vi "LoadConfig.vi"(8 "error in (no error)":errorcluster, 11 "EpiWrapper in":refnum<class "EpiWrapper.lvclass">) -> (0 "error out":errorcluster, 3 "EpiWrapper out":refnum<class "EpiWrapper.lvclass">)   [LabVIEW 2012, in "EpiWrapper.lvclass"]
uses:
  EpiWrapper.lvclass
  <vilib>/xml/Load XML File.vi
  <vilib>/xml/Close Reference(Node).vi
  <vilib>/xml/Close Reference(NdList).vi
  <resource>/objmgr/DOMUserDefRef.rc
  <vilib>/xml/NI_XML.lvlib
panel:
  out "Array":cluster{"IntTime":string, "Samples":string}[](array[cluster])
  out "Parse Errors":string
  out "XML File Path":path
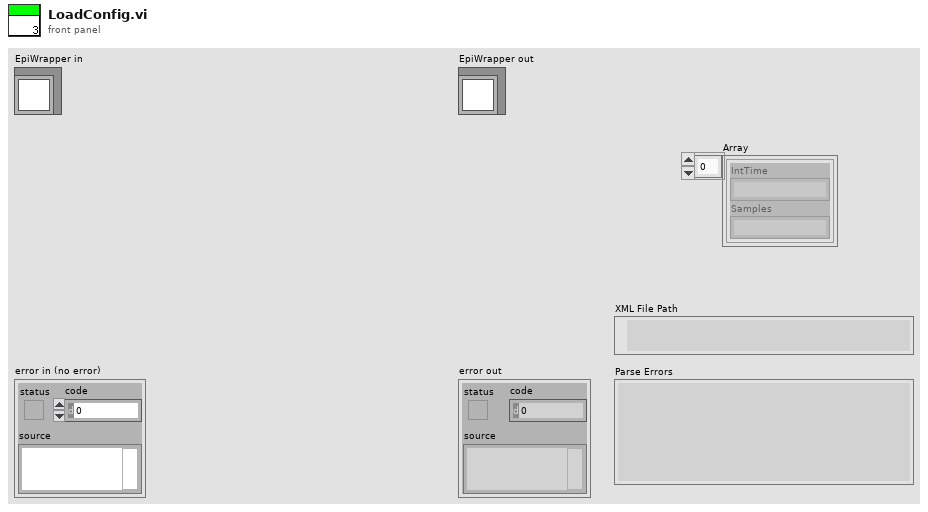
[diagram p1: front panel]
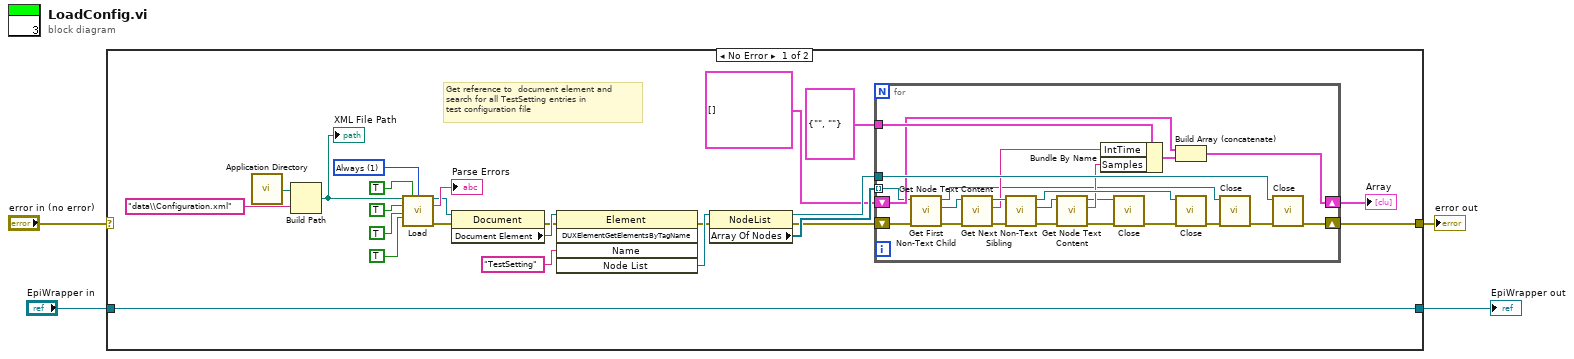
[diagram p0: block diagram]
diagram:
  n1 = case shown="No Error" "error in (no error)" {
    selector: "error in (no error)" -> [_ w53]
    tunnel: "EpiWrapper in" -> [w5 w52]
    tunnel: [w7 w53] -> w2
    tunnel: [w5 w52] -> w1
    frame No Error {
      w25 = 1 items=["Never", "Always", "Auto"] ("Validate On Load")
      # "Get reference to  document element and\nsearch for all TestSetting entries in \ntest configuration file"
      n2 = call <vilib>:"Application Directory.vi"() -> ("Application Directory"=w6:path)
      n3 = Build Path(base path=w6, name or relative path="data\\Configuration.xml") -> (appended path=w15:path)
      "XML File Path" <- w15
      n4 = call-poly <vilib>:"Load.vi"("path to XML document"=w15, "preserve whitespace (True)"=TRUE ("Preserve Whitespace"), "validate on load (Auto)"=w25, "process namespaces (False)"=TRUE ("Do Namespaces"), "process schema (False)"=TRUE ("Do Schema"), "load external DTD (True)"=TRUE ("Load External DTD")) -> ("DOM document out"=w17:refnum<k20>, "parse errors"=→"Parse Errors":string, "error out"=w16:errorcluster)  [unwired: 1 in, 6 out]
      n5 = property class="Document"(reference=w17, error in=w16) -> (error out=w20:errorcluster, "Document Element"=w21:refnum<k20>)  [unwired: 1 out]
      n6 = invoke class="Element" method="DUXElementGetElementsByTagName"(reference=w21, error in=w20, "Name"="TestSetting" ("Node Name")) -> (error out=w18:errorcluster, "Node List"=w19:refnum<k20>)  [unwired: 2 in, 3 out]
      n7 = property class="NodeList"(reference=w19, error in=w18) -> (reference out=w13:refnum<k20>, error out=w8:errorcluster, "Array Of Nodes"=w12:refnum<k20>[])
      n8 = for {
        tunnel: w12 -> [w32] mode=indexing
        tunnel: w13 -> [w42]
        shift-right: [w35] -> w9
        shift-left: cluster{"IntTime":string, "Samples":string}[] [] -> [w37]
        shift-right: [w41] -> w7
        shift-left: w8 -> [w34]
        tunnel: cluster{"IntTime":string, "Samples":string} {"IntTime"="", "Samples"=""} -> [w40]
        n9 = call <vilib>:"Get First Non-Text Child.vi"("error in (no error)"=w34, "node in"=w32) -> ("error out"=w50:errorcluster, "child node"=w51:refnum<k20>, "node out"=w29:refnum<k20>)  [unwired: 7 out]
        n10 = call <vilib>:"Get Node Text Content.vi"("error in (no error)"=w50, "node in"=w51) -> ("error out"=w46:errorcluster, "node text"=w39:string, "node out"=w47:refnum<k20>)  [unwired: 7 out]
        n11 = call <vilib>:"Get Next Non-Text Sibling.vi"("error in (no error)"=w46, "node in"=w47) -> ("error out"=w49:errorcluster, "sibling node"=w48:refnum<k20>, "node out"=w45:refnum<k20>)  [unwired: 7 out]
        n12 = call <vilib>:"Get Node Text Content.vi"("error in (no error)"=w49, "node in"=w48) -> ("error out"=w30:errorcluster, "node text"=w38:string, "node out"=w31:refnum<k20>)  [unwired: 7 out]
        n13 = Bundle By Name(cluster=w40, "IntTime"=w39, "Samples"=w38) -> (w36:cluster{"IntTime":string, "Samples":string})
        n14 = call-poly <vilib>:"Close.vi"("error in (no error)"=w30, "node"=w31) -> ("error out"=w44:errorcluster)  [unwired: 7 out]
        n15 = Build Array (concatenate)(w37, w36) -> (w35:cluster{"IntTime":string, "Samples":string}[])
        n16 = call-poly <vilib>:"Close.vi"("error in (no error)"=w44, "node"=w45) -> ("error out"=w43:errorcluster)  [unwired: 7 out]
        n17 = call-poly <vilib>:"Close.vi"("error in (no error)"=w43, "node"=w29) -> ("error out"=w33:errorcluster)  [unwired: 7 out]
        n18 = call-poly <vilib>:"Close.vi"("error in (no error)"=w33, "node list"=w42) -> ("error out"=w41:errorcluster)  [unwired: 7 out]
      }
      "Array" <- w9
    }
    frame Error {
    }
  }
  "error out" <- w2
  "EpiWrapper out" <- w1
